vi "cRIO_FPGA_COMMUNICATION  Get Data from Specific Station.vi"(8 "Fehler (Eingang, kein Fehler)":errorcluster, 10 "Station Index":T1, 11 "Stationen (Daten einer Station pro Spalte)":u16[][](array[numeric])) -> (0 "Fehler (Ausgang)":errorcluster, 2 "Station Data":bool[][](array[boolean]), 3 "Band Data":bool[][](array[boolean]))   [LabVIEW 2013, in "cRIO_FPGA_COMMUNICATION.lvlib"]
uses:
  cRIO_FPGA_COMMUNICATION.lvlib
  TYPES/TYPE Station Index.ctl
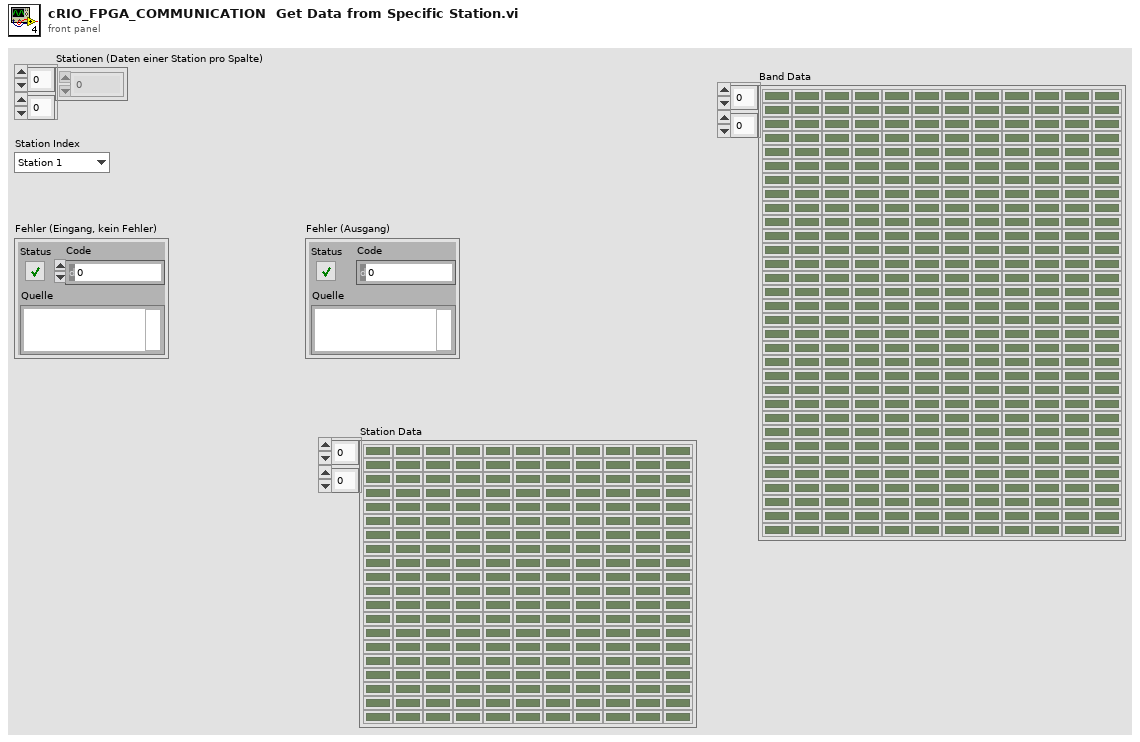
[diagram p1: front panel]
types:
  T1 = typedef "cRIO_FPGA_COMMUNICATION.lvlib/TYPE Station Index.ctl" = enum16{"Station 1", "Station 2", "Station 3", "Station 4", "Station 5", "Station 6", "Station 7", "Station 8", "Station 9", "Station 10", "Station 11", "Station 12", "Station 13", "Station 14", "Station 15", "Station 16", "Station 17", "Station 18", "Station 19", "Station 20"}
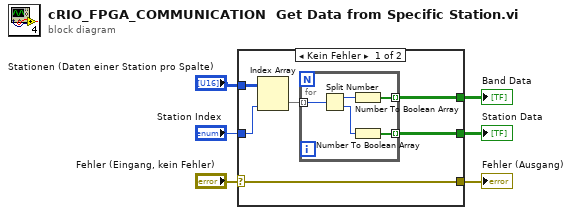
[diagram p0: block diagram]
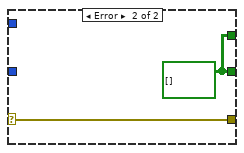
[diagram p2: hidden frame]
diagram:
  n1 = case shown="Kein Fehler" "Fehler (Eingang, kein Fehler)" {
    selector: "Fehler (Eingang, kein Fehler)" -> [w7 w18]
    tunnel: "Stationen (Daten einer Station pro Spalte)" -> [w12 _]
    tunnel: "Station Index" -> [w11 _]
    tunnel: [w9 w19] -> w3
    tunnel: [w8 w19] -> w4
    tunnel: [w7 w18] -> w6
    frame No Error {
      n2 = Index Array(array=w12, index (col)=w11) -> (element=w10:u16[])  [unwired: 1 in]
      n3 = for {
        tunnel: w10 -> [w17] mode=indexing
        tunnel: [w14] -> w9 mode=indexing
        tunnel: [w13] -> w8 mode=indexing
        n4 = Split Number(x=w17) -> (hi(x)=w16:u8, lo(x)=w15:u8)
        n5 = Number To Boolean Array(number=w16) -> (Boolean array=w14:bool[])
        n6 = Number To Boolean Array(number=w15) -> (Boolean array=w13:bool[])
      }
    }
    frame Error {
      w19 = bool[][] [] ("Boolean array")
    }
  }
  "Fehler (Ausgang)" <- w6
  "Station Data" <- w4
  "Band Data" <- w3
